vi "Enable Charge Pump.vi"(8 "Error In":errorcluster, 11 "LINX Resource":T1) -> (0 "Error Out":errorcluster, 3 "LINX Resource":T1)   [LabVIEW 2020, in "LMH-LINX.lvlib" / "SSD1306.lvlib"]
doc: "Enabled the SSD1306's internal charge pump."
uses:
  SSD1306.lvlib
  Private/Type Defs/LINX Ref.ctl
  Private/Type Defs/Platform.ctl
  Private/Type Defs/Interface.ctl
  Private/Device/Type Defs/LINX Device Config.ctl
  Private/Device/Type Defs/TCP Config.ctl
  Private/Device/Type Defs/Channels.ctl
  Private/SSD1306 FGV State.ctl
  Peripherals/SPI/SPI CS Config.ctl
  Private/Type Defs/Peripherals/SPI/SPI CS Logic Level.ctl
  Peripherals/Digital/Digital Write 1 Chan.vi
  Peripherals/SPI/SPI Write Read 1 Frame.vi
  Peripherals/Digital/Digital Write N Chans.vi
  Peripherals/SPI/SPI Write Read N Frames.vi
  Private/Local IO/LinxDigitalWrite.vi
  Utilities/Check Channel.vi
  Private/Local IO/LinxSpiWriteRead.vi
  Private/Utilties/Generate Error.vi
  LMH-LINX.lvlib
  Private/Device/Device.lvlib
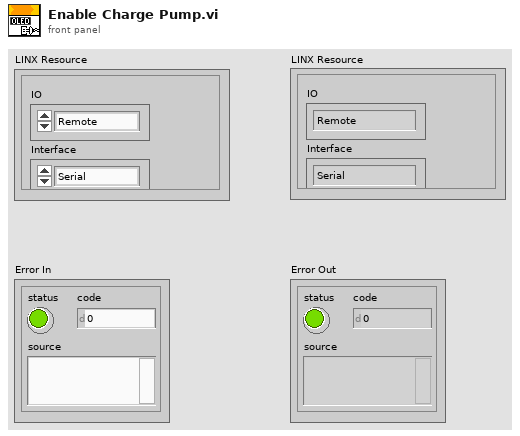
[diagram p1: front panel]
types:
  T1 = typedef "LMH-LINX.lvlib/LINX Ref.ctl" = cluster{"IO":T2, "Interface":T3, "LINX Device Config":T4}
  T2 = typedef "LMH-LINX.lvlib/Platform.ctl" = enum16{"Remote", "Local"}
  T3 = typedef "LMH-LINX.lvlib/Interface.ctl" = enum16{"Serial", "TCP"}
  T4 = typedef "LMH-LINX.lvlib/Device.lvlib/LINX Device Config.ctl" = cluster{"Interface":T3, "COM Port":refnum<visa-resource-name>, "TCP Configuration":T5, "Device Family":u8, "Device ID":u8, "Device Name":string, "TCP Ref":refnum<k5>, "Channels":T6}
  T5 = typedef "LMH-LINX.lvlib/Device.lvlib/TCP Config.ctl" = cluster{"IP Address":string, "Port":u16}
  T6 = typedef "LMH-LINX.lvlib/Channels.ctl" = cluster{"DI":u8[], "DO":u8[], "AI":u8[], "AO":u8[], "PWM":u8[], "QE":u8[], "UART":u8[], "I2C 2":u8[], "SPI":u8[], "CAN":u8[], "Servo":u8[], "AI Ref (V)":dbl, "AI Resolution (Bits)":u8, "AO Ref (V)":dbl, "AO Resolution (Bits)":u8}
  T7 = typedef "LMH-LINX.lvlib/SPI CS Config.ctl" = cluster{"CS Channel":u8, "CS Logic Level":T8}
  T8 = typedef "LMH-LINX.lvlib/SPI CS Logic Level.ctl" = enum8{"Active Low", "Active High"}
  T9 = typedef "LMH-LINX.lvlib/SSD1306.lvlib/SSD1306 FGV State.ctl" = enum16{"Init", "Set", "Get"}
  T10 = typedef "LMH-LINX.lvlib/SSD1306.lvlib/SSD1306 Config.ctl" = cluster{"SPI Channel (0)":u8, "VDD Channel":u8, "VBAT Channel":u8, "RESET Channel":u8, "DC Channel":u8, "SPI CS (3)":u8}
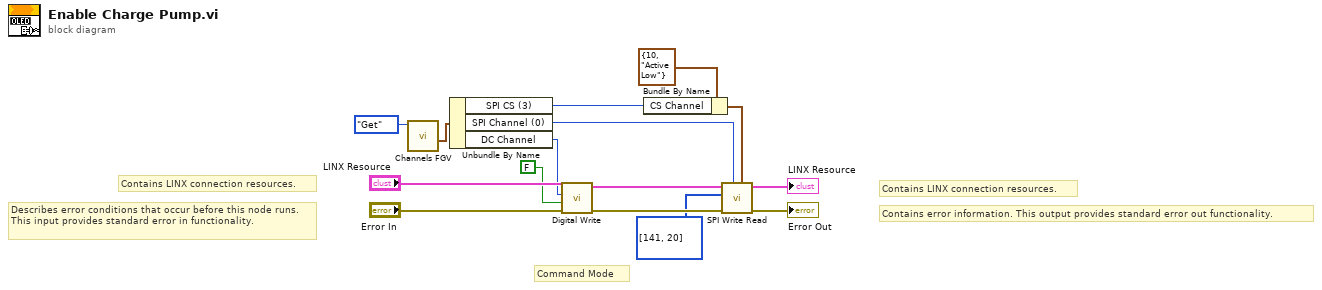
[diagram p0: block diagram]
diagram:
  # "Contains LINX connection resources."
  # "Contains error information. This output provides standard error out functionality."
  # "Contains LINX connection resources."
  # "Describes error conditions that occur before this node runs. This input provides standard error in functionality."
  # "Command Mode"
  n1 = call "Channels FGV.vi"("SSD1306 FGV State"=SSD1306_FGV_State."Get") -> ("SSD1306 Channels"=w12:T10)  [unwired: 10 in]
  n2 = Unbundle By Name(w12) -> ("SPI CS (3)"=w3:u8, "SPI Channel (0)"=w1:u8, "DC Channel"=w11:u8)
  n3 = call-poly "Digital Write.vi"("Error In"="Error In", "Output Value"=FALSE, "DO Channel"=w11, "LINX Resource"="LINX Resource") -> ("Error Out"=w7:errorcluster, "LINX Resource"=w9:T1)  [unwired: 6 in]
  n4 = Bundle By Name(cluster=T7 {"CS Channel"=10, "CS Logic Level"=enum."Active Low"} ("CS Configuration"), "CS Channel"=w3) -> (w2:T7)
  n5 = call-poly "SPI Write Read.vi"("CS Configuration"=w2, "SPI Channel (0)"=w1, "Error In"=w7, "Data"=u8[] [141, 20], "LINX Resource"=w9) -> ("Error Out"=→"Error Out":errorcluster, "LINX Resource"=→"LINX Resource":T1)  [unwired: 3 in, 2 out]
